vi "ASK_16_Point to Point.vi"() -> ()   [LabVIEW 2015]
uses:
  <instrlib>/niUSRP/niUSRP Write Tx Data (CDB).vi
panel:
  out "Waveform Graph":dbl[](graph)
  out "error out":errorcluster
  out "coerced IQ rate":dbl=100000.0 format="%#_6p"
  out "coerced carrier frequency":dbl=100000.0 format="%#_6p"
  out "coerced gain":dbl format="%#_6f"
  in  "IQ rate":dbl=100000.0 format="%#_6p"
  in  "carrier frequency":dbl=100000.0 format="%#_6p"
  in  "gain":dbl format="%#_6f"
  in  "active antenna":string
  in  "device names":refnum<k15>
  in  "y":bool
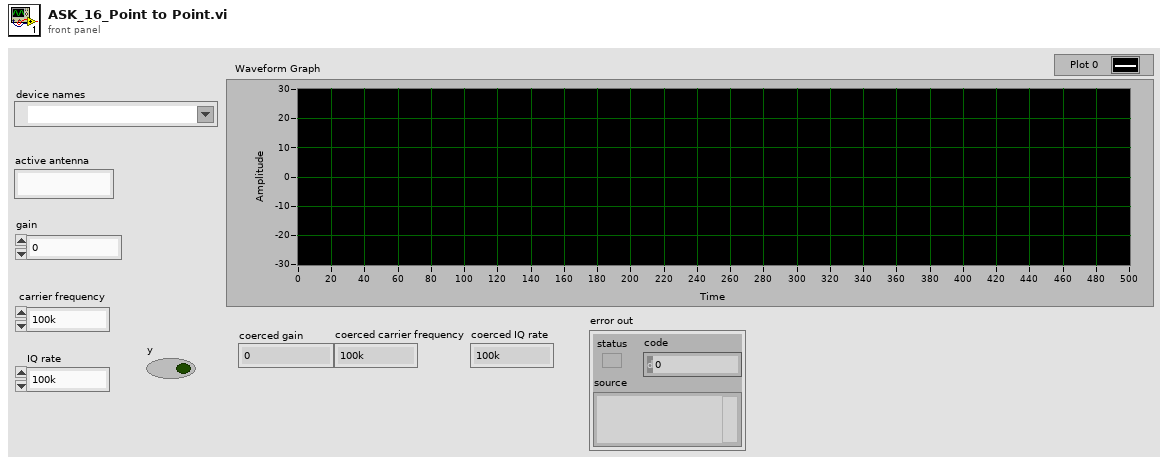
[diagram p1: front panel]
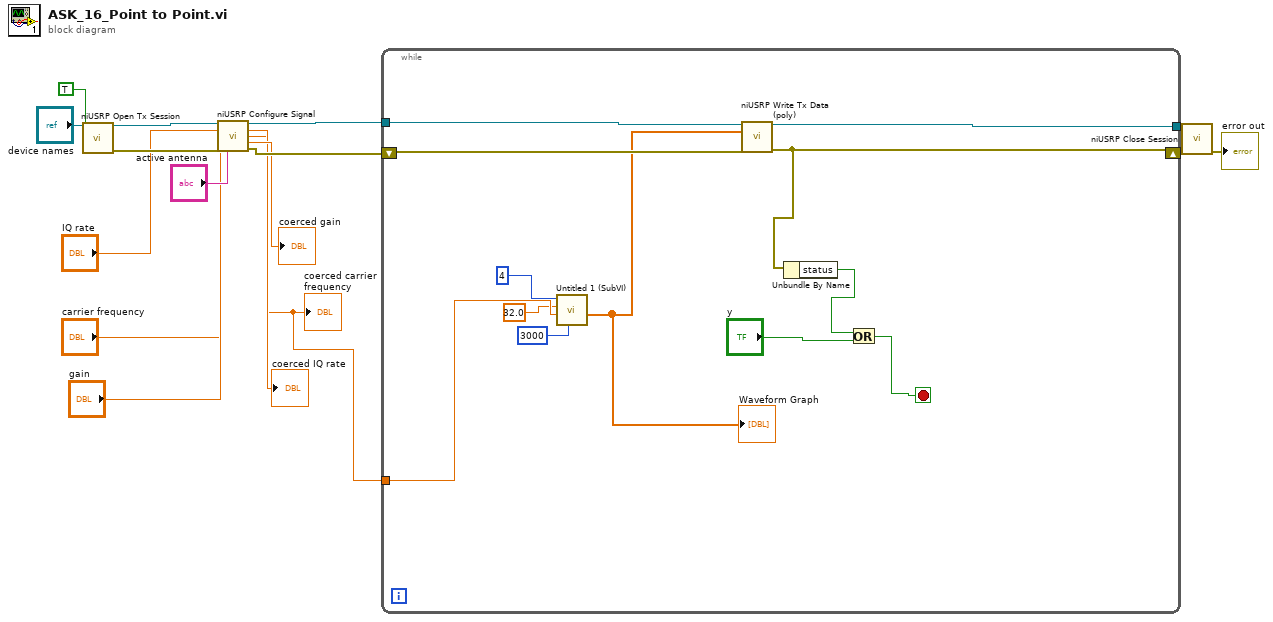
[diagram p0: block diagram]
diagram:
  n1 = call <instrlib>:"niUSRP Open Tx Session.vi"("device names"="device names", "reset"=TRUE) -> ("session handle out"=w15:refnum<k15>, "error out"=w14:errorcluster)  [unwired: 12 in]
  n2 = call <instrlib>:"niUSRP Configure Signal.vi"("session handle"=w15, "IQ rate"="IQ rate", "carrier frequency"="carrier frequency", "gain"="gain", "error in (no error)"=w14, "active antenna"="active antenna") -> ("session handle out"=w5:refnum<k15>, "coerced IQ rate"=→"coerced IQ rate":dbl, "coerced carrier frequency"=w1:dbl, "coerced gain"=→"coerced gain":dbl, "error out"=w8:errorcluster)  [unwired: 5 in]
  "coerced carrier frequency" <- w1
  n3 = while {
    shift-right: [w25] -> w4
    shift-left: w8 -> [w28]
    tunnel: w5 -> [w27]
    tunnel: [w26] -> w3
    tunnel: w1 -> [w21]
    stop <- w22 stop-if-true
    n4 = call "Untitled 1 (SubVI).vi"("Sampling freq."=3000, "Carrier Frequency"=w21, "number of bits"=32.0, "Number of Cycles"=4) -> ("output"=w17:dbl[])  [unwired: 3 in, 4 out]
    "Waveform Graph" <- w17
    n5 = call-poly <instrlib>:"niUSRP Write Tx Data (poly).vi"("session handle"=w27, "data"=w17, "error in (no error)"=w28) -> ("session handle out"=w26:refnum<k15>, "error out"=w25:errorcluster)  [unwired: 11 in]
    n6 = Unbundle By Name(w25) -> ("status"=w24:bool)
    n7 = Or(x=w24, y="y") -> (x .or. y?=w22:bool)
  }
  n8 = call <instrlib>:"niUSRP Close Session.vi"("session handle"=w3, "error in (no error)"=w4) -> ("error out"=→"error out":errorcluster)  [unwired: 13 in]
